vi "Setposition.vi"(8 "error in":errorcluster, 11 "Position[µm]":dbl format="%#_13g") -> (0 "error out":errorcluster)   [LabVIEW 2015]
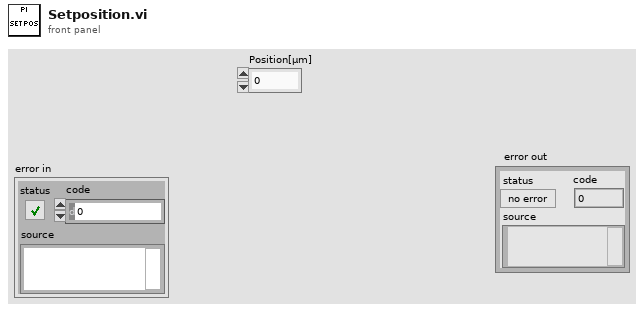
[diagram p1: front panel]
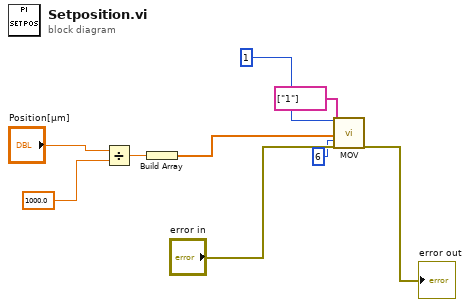
[diagram p0: block diagram]
diagram:
  n1 = Divide(x="Position[µm]", y=1000.0) -> (x/y=w2:dbl)
  n2 = Build Array(w2) -> (w5:dbl[])
  n3 = call "MOV.vi"("System no."=1, "Axes to move"=string[] ["1"], "Position values"=w5, "No.of digits"=i16 6, "error in"="error in") -> ("error out"=→"error out":errorcluster)  [unwired: 14 out]
